vi "Get_Open_LV_Files.vi"(8 "error in (no error)":errorcluster, 11 "Items to be ignored":string[](array[string])) -> (0 "error out":errorcluster, 2 "Application:All VIs In Memory":string[](array[string]))   [LabVIEW 2013]
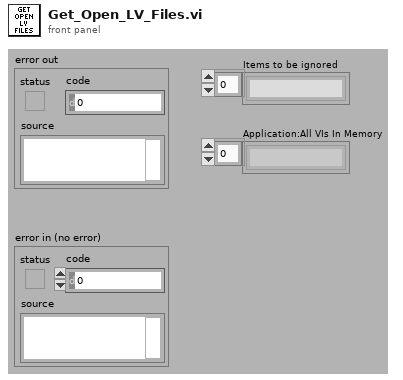
[diagram p1: front panel]
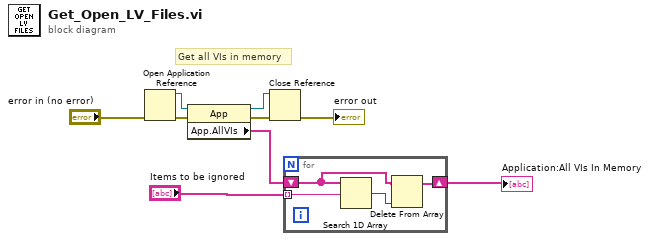
[diagram p0: block diagram]
diagram:
  # "Get all VIs in memory"
  n1 = Open Application Reference(8:"error in (no error)") -> (0:w5:errorcluster, 3:w8:refnum<vi>)  [unwired: 3 in]
  n2 = property class="App"(reference=w8, error in=w5) -> (reference out=w9:refnum<vi>, error out=w4:errorcluster, "App.AllVIs"=w2:string[])
  n3 = Close Reference(reference=w9, error in (no error)=w4) -> (error out=→"error out":errorcluster)
  n4 = for {
    tunnel: "Items to be ignored" -> [w13] mode=indexing
    shift-right: [w11] -> w3
    shift-left: w2 -> [w12]
    n5 = Search 1D Array(1D array=w12, element=w13) -> (index of element=w10:i32)  [unwired: 1 in]
    n6 = Delete From Array(array=w12, index=w10) -> (array with subset deleted=w11:string[])  [unwired: 1 in, 1 out]
  }
  "Application:All VIs In Memory" <- w3
